vi "AxisFetchConf.vi"(8 "error in":errorcluster, 11 "Modbus master":refnum<class "Modbus Master.lvclass">) -> (0 "error out":errorcluster, 2 "JoyControl":T1 {"UnitsControl" items=["mm", "°"]}, 3 "AxisConfiguration":T2={"AxisHomeType"=1, "AxisBacklash"=0.0, "AxisGain"=1.0, "AxisOffset"=0.0, "AxisUnit"=1, "ReqConfRead"=FALSE, "ReqConfWrite"=FALSE, "AxisName"="", "AxisAccDecc"=0.0, "AxisHomeVel"=0.0} {"AxisUnit" items=["mm", "°"]; "AxisHomeType" items=["no homing"=0, "forward limit switch"=1, "backward limit switch"=2, "forward reference"=4, "backward reference"=8]})   [LabVIEW 2020, in "SMCD14_lib.lvlib"]
uses:
  SMCD14_lib.lvlib
  <vilib>/Modbus/master/Modbus Master.lvclass
  AxisConfiguration_typedef.ctl
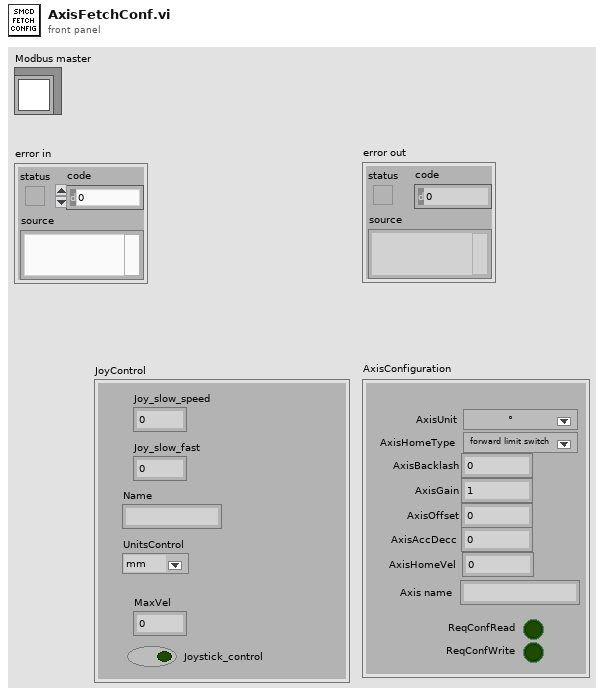
[diagram p1: front panel]
types:
  T1 = cluster{"Joy_slow_speed":sgl, "Joy_slow_fast":sgl, "Name":string, "UnitsControl":u16, "MaxVel":sgl, "Joystick_control":bool}
  T2 = typedef "SMCD14_lib.lvlib/AxisConfiguration_typedef.ctl" = cluster{"AxisHomeType":u16, "AxisBacklash":dbl, "AxisGain":dbl, "AxisOffset":dbl, "AxisUnit":u16, "ReqConfRead":bool, "ReqConfWrite":bool, "AxisName":string, "AxisAccDecc":dbl, "AxisHomeVel":dbl}
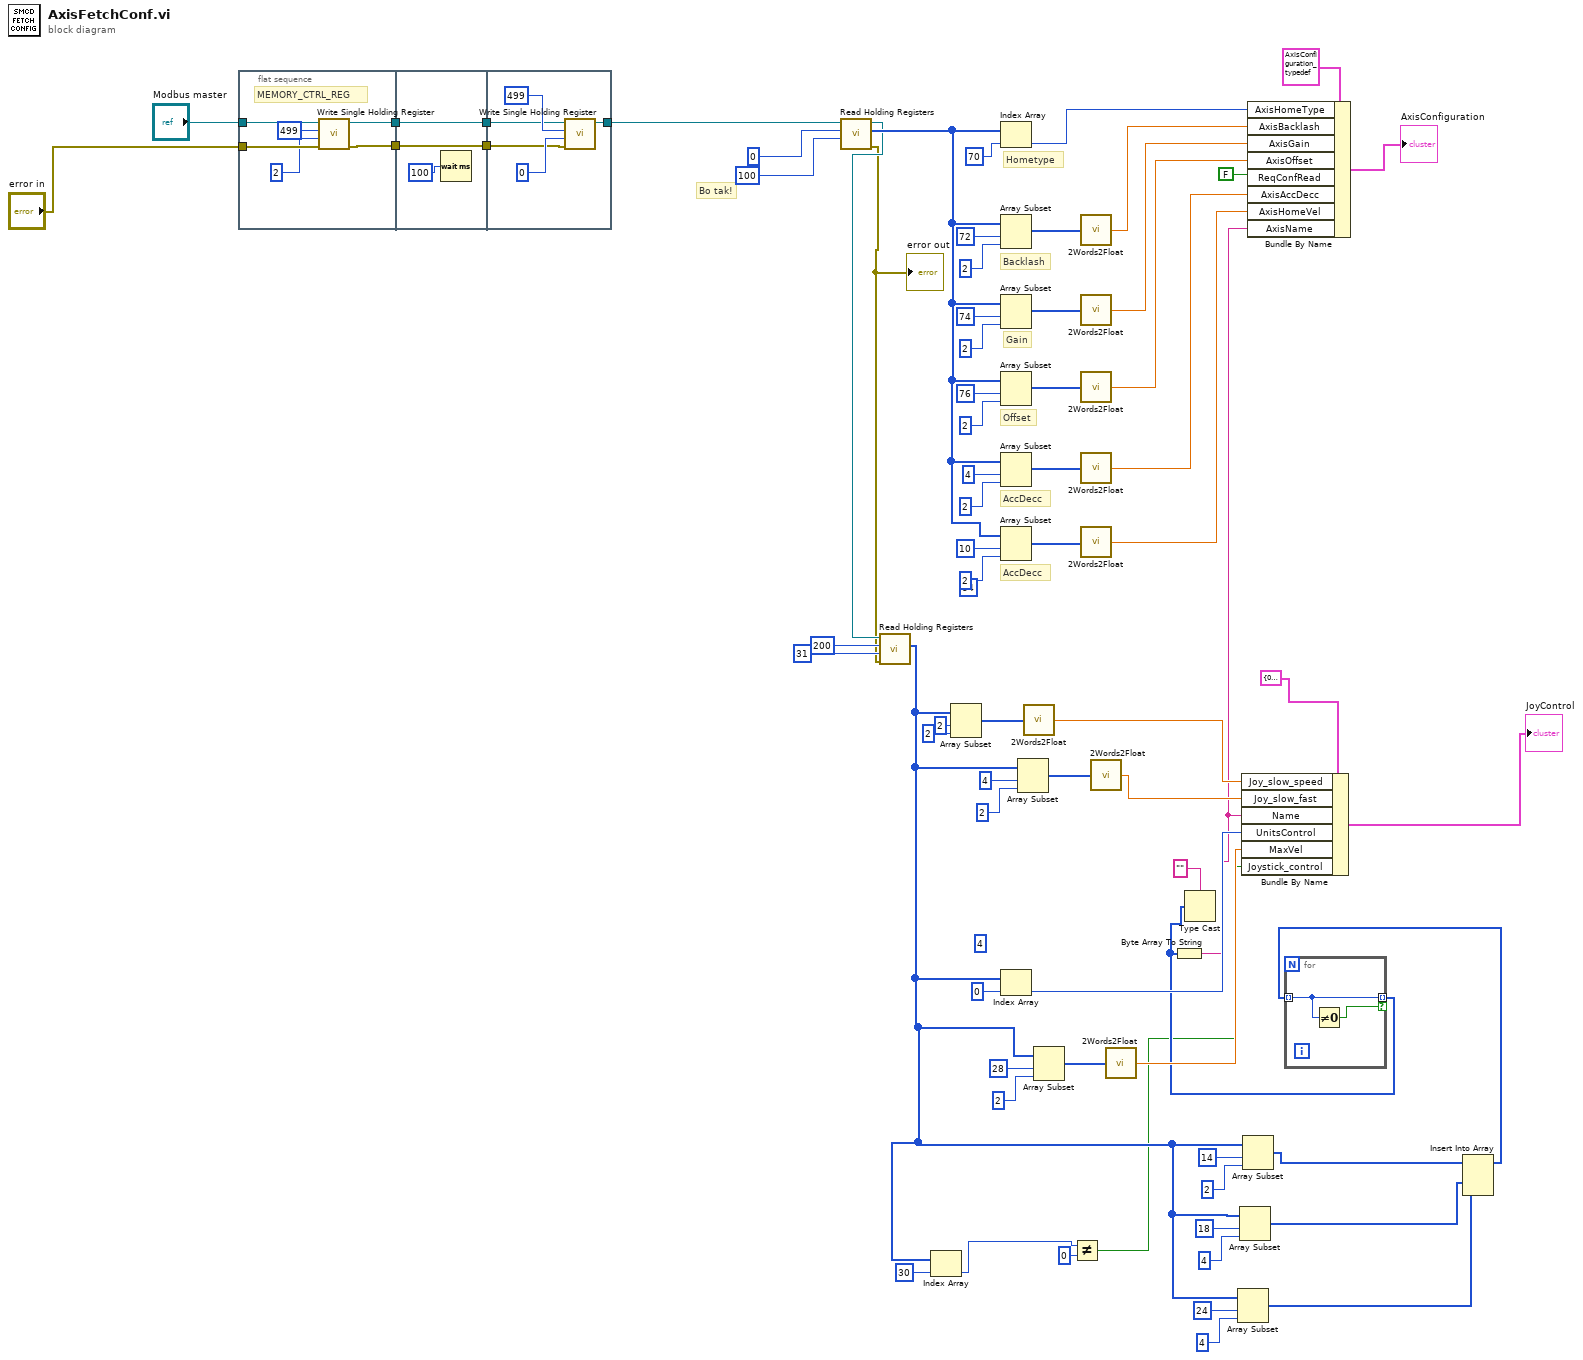
[diagram p0: block diagram]
diagram:
  (unwired) 4 ("length")
  (unwired) 34 ("index")
  # "AccDecc"
  # "AccDecc"
  # "Bo tak!"
  # "Offset"
  # "Gain"
  # "Backlash"
  # "Hometype"
  n1 = flat-sequence {
    tunnel: "Modbus master" -> [w79]
    tunnel: "error in" -> [w77]
    tunnel: [w78] -> w47
    tunnel: [w74] -> w45
    tunnel: w47 -> [w82]
    tunnel: [w82] -> w46
    tunnel: w45 -> [w80]
    tunnel: [w80] -> w44
    tunnel: [w83] -> w49
    tunnel: w46 -> [w85]
    tunnel: w44 -> [w84]
    frame #0 {
      # "MEMORY_CTRL_REG"
      n2 = call-dynamic "Write Single Holding Register.vi"("error in (no error)"=w77, "holding register value"=u16 2, "address"=u16 499, "Modbus master in"=w79) -> ("error out"=w74:errorcluster, "Modbus master out"=w78:refnum<class "Modbus Master.lvclass">)  [unwired: 6 in]
    }
    frame #1 {
      n3 = Wait (ms)(milliseconds to wait=u32 100) -> ()  [unwired: 1 out]
    }
    frame #2 {
      n4 = call-dynamic "Write Single Holding Register.vi"("error in (no error)"=w84, "holding register value"=u16 0, "address"=u16 499, "Modbus master in"=w85) -> ("Modbus master out"=w83:refnum<class "Modbus Master.lvclass">)  [unwired: 6 in, 1 out]
    }
  }
  n5 = call-dynamic "Read Holding Registers.vi"("number of holding registers"=u16 100, "starting address"=u16 0, "Modbus master in"=w49) -> ("error out"=w20:errorcluster, "register values"=w41:u16[], "Modbus master out"=w21:refnum<class "Modbus Master.lvclass">)  [unwired: 6 in]
  "error out" <- w20
  n6 = call-dynamic "Read Holding Registers.vi"("error in (no error)"=w20, "number of holding registers"=u16 31, "starting address"=u16 200, "Modbus master in"=w21) -> ("register values"=w3:u16[])  [unwired: 5 in, 2 out]
  n7 = Index Array(array=w3, index=30) -> (element=w4:u16)
  n8 = Array Subset(array=w3, index=2, length=2) -> (w34:u16[])
  n9 = Index Array(array=w41, index=70) -> (element=w70:u16)
  n10 = Array Subset(array=w41, index=72, length=2) -> (w67:u16[])
  n11 = Array Subset(array=w41, index=74, length=2) -> (w63:u16[])
  n12 = Array Subset(array=w41, index=76, length=2) -> (w60:u16[])
  n13 = Array Subset(array=w41, index=4, length=2) -> (w54:u16[])
  n14 = Array Subset(array=w41, index=10, length=2) -> (w40:u16[])
  n15 = Index Array(array=w3, index=0) -> (element=w26:u16)
  n16 = Array Subset(array=w3, index=4, length=2) -> (w30:u16[])
  n17 = call "2Words2Float.vi"("input"=w34) -> ("value"=w33:sgl)
  n18 = Array Subset(array=w3, index=28, length=2) -> (w23:u16[])
  n19 = Not Equal?(x=w4, y=u16 0) -> (x != y?=w2:bool)
  n20 = call "2Words2Float.vi"("input"=w67) -> ("value"=w66:sgl)
  n21 = call "2Words2Float.vi"("input"=w63) -> ("value"=w59:sgl)
  n22 = call "2Words2Float.vi"("input"=w60) -> ("value"=w58:sgl)
  n23 = call "2Words2Float.vi"("input"=w54) -> ("value"=w51:sgl)
  n24 = call "2Words2Float.vi"("input"=w40) -> ("value"=w39:sgl)
  n25 = call "2Words2Float.vi"("input"=w30) -> ("value"=w29:sgl)
  n26 = call "2Words2Float.vi"("input"=w23) -> ("value"=w22:sgl)
  n27 = Array Subset(array=w3, index=24, length=4) -> (w10:u16[])
  n28 = Array Subset(array=w3, index=18, length=4) -> (w11:u16[])
  n29 = Array Subset(array=w3, index=14, length=2) -> (w12:u16[])
  n30 = Insert Into Array(array=w12, new element #1=w11, new element #2=w10) -> (w9:u16[])  [unwired: 1 in]
  n31 = for {
    tunnel: w9 -> [w88] mode=indexing
    tunnel: [w88] -> w8 mode=indexing if=w89
    n32 = Not Equal To 0?(x=w88) -> (x != 0?=w89:bool)
  }
  n33 = Byte Array To String(unsigned byte array=w8) -> (string=w1:string)
  n34 = Type Cast(type="", x=w8) -> ()  [unwired: 1 out]
  n35 = Bundle By Name(cluster=T1 {"Joy_slow_speed"=0.0, "Joy_slow_fast"=0.0, "Name"="", "UnitsControl"=0, "MaxVel"=0.0, "Joystick_control"=FALSE} ("JoyControl"), "Joy_slow_speed"=w33, "Joy_slow_fast"=w29, "Name"=w1, "UnitsControl"=w26, "MaxVel"=w22, "Joystick_control"=w2) -> (→"JoyControl":T1)
  n36 = Bundle By Name(cluster=T2 {"AxisHomeType"=4, "AxisBacklash"=0.699999988079071, "AxisGain"=6.0, "AxisOffset"=0.0, "AxisUnit"=0, "ReqConfRead"=FALSE, "ReqConfWrite"=FALSE, "AxisName"="", "AxisAccDecc"=0.0, "AxisHomeVel"=0.0} ("AxisConfiguration"), "AxisHomeType"=w70, "AxisBacklash"=w66, "AxisGain"=w59, "AxisOffset"=w58, "ReqConfRead"=FALSE, "AxisAccDecc"=w51, "AxisHomeVel"=w39, "AxisName"=w1) -> (→"AxisConfiguration":T2)
